vi "例4-32.vi"() -> ()   [LabVIEW 2019]
panel:
  out "强度图表":dbl[][](graph)
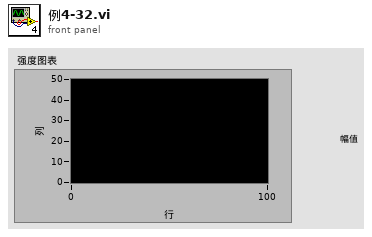
[diagram p1: front panel]
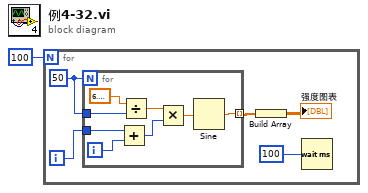
[diagram p0: block diagram]
diagram:
  n1 = for {
    N: 100 -> [_]
    i -> [w5]
    w6 = 50
    n2 = for {
      N: w6 -> [_]
      tunnel: w6 -> [w12]
      tunnel: w5 -> [w10]
      tunnel: [w7] -> w4 mode=indexing
      i -> [w11]
      n3 = Add(x=w10, y=w11) -> (x+y=w9:i32)
      n4 = Divide(x=6.283185307179586, y=w12) -> (x/y=w14:dbl)
      n5 = Multiply(x=w14, y=w9) -> (x*y=w8:dbl)
      n6 = Sine(x=w8) -> (sin(x)=w7:dbl)
    }
    n7 = Build Array(w4) -> (→"强度图表":dbl[][])
    n8 = Wait (ms)(milliseconds to wait=100) -> ()  [unwired: 1 out]
  }
